vi "Fake System Time Stamp.vi"() -> ()   [LabVIEW 2009]
panel:
  in  "Time Stamp":timestamp
  in  "background":dbl format="%<%I:%M:%S %p\n%m/%d/%Y>T"
  # "There are two controls here, grouped. The front control is a Classic time stamp, which is the control you operate on.\nThe control behind it is a System numeric, which is just providing decoration."
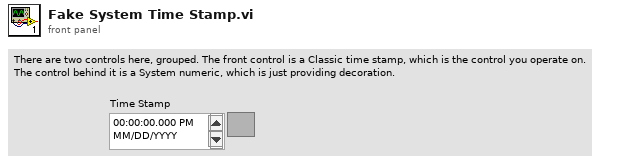
[diagram p1: front panel]
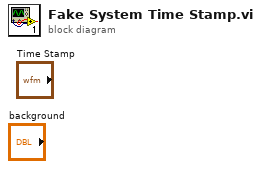
[diagram p0: block diagram]
diagram:
